vi "LockinGPIB.vi"(7 "P-LockIn":string="23", 8 "error in (no error)":errorcluster, 9 "delay":i32=1000 min=100 max=3000, 10 "Num. Lect":i32=1 min=1 max=20) -> (0 "error out":errorcluster, 2 "LockIn":dbl=-0.0002)   [LabVIEW 2018]
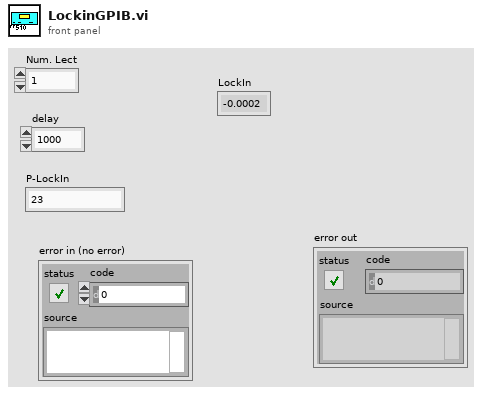
[diagram p1: front panel]
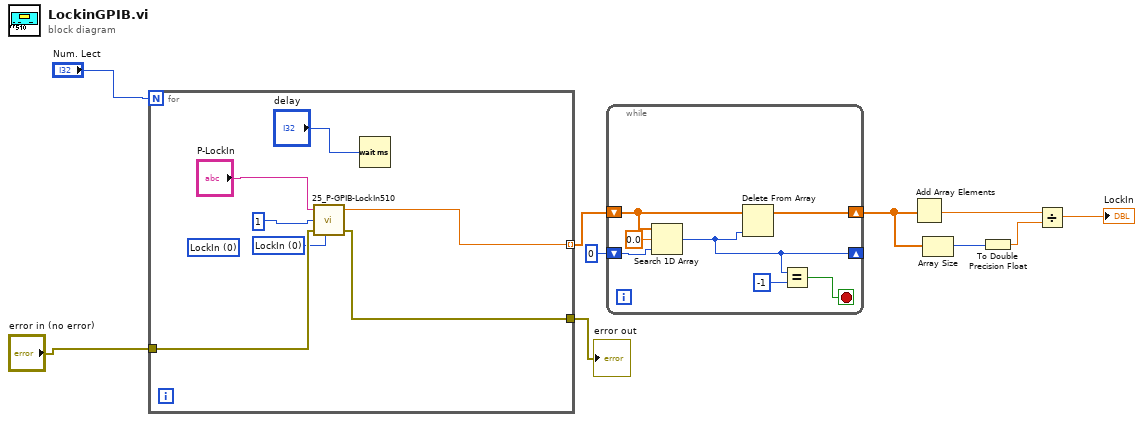
[diagram p0: block diagram]
diagram:
  n1 = for {
    N: "Num. Lect" -> [_]
    tunnel: [w11] -> w3 mode=indexing
    tunnel: "error in (no error)" -> [w16]
    tunnel: [w15] -> w4
    w14 = u16 0 items=["LockIn", "LockIn-DMM"] ("Tipo")
    (unwired) u16 0 items=["LockIn", "LockIn-DMM"] ("Tipo")
    n2 = call "25_P-GPIB-LockIn510.vi"("P-LockIn"="P-LockIn", "Lecturas"=1, "error in (no error)"=w16, "Tipo"=w14) -> ("LockIn"=w11:dbl, "error out"=w15:errorcluster)  [unwired: 1 in, 1 out]
    n3 = Wait (ms)(milliseconds to wait="delay") -> ()  [unwired: 1 out]
  }
  "error out" <- w4
  n4 = while {
    shift-right: [w22] -> w2
    shift-left: w3 -> [w23]
    shift-right: [w20] -> _
    shift-left: 0 ("index of element") -> [w21]
    stop <- w18 stop-if-true
    n5 = Search 1D Array(1D array=w23, element=0.0, start index (0)=w21) -> (index of element=w20:i32)
    n6 = Delete From Array(array=w23, index=w20) -> (array with subset deleted=w22:dbl[])  [unwired: 1 in, 1 out]
    n7 = Equal?(x=w20, y=-1) -> (x = y?=w18:bool)
  }
  n8 = Add Array Elements(numeric array=w2) -> (sum=w9:dbl)
  n9 = Array Size(array=w2) -> (size(s)=w8:i32)
  n10 = To Double Precision Float(number=w8) -> (double precision float=w7:dbl)
  n11 = Divide(x=w9, y=w7) -> (x/y=→"LockIn":dbl)
